vi "ST Step Joint.vi"(5 "error in (no error)":errorcluster, 6 "STEPS":string="1000", 7 "Combo Box":string(combo)="WAIST", 8 "VISA resource name":refnum<visa-resource-name>) -> (0 "error out":errorcluster, 1 "String Received":string, 2 "Ready and OK":bool, 3 "VISA resource name out":refnum<visa-resource-name>, 4 "Result Code":i32)   [LabVIEW 2009]
doc: "This VI will rotate a single joint, using joint mode. Select the joint to be rotated and the number of motor steps, - indicates reverse."
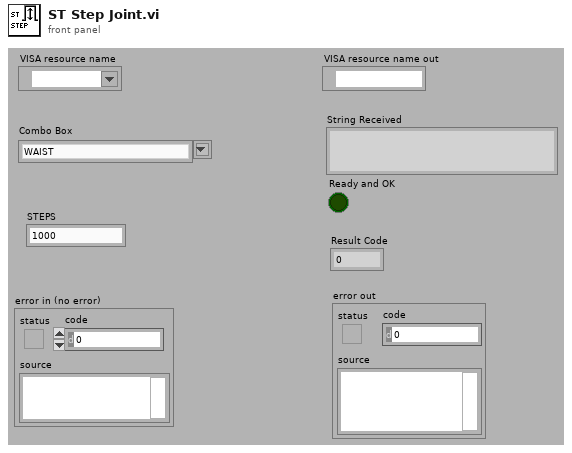
[diagram p1: front panel]
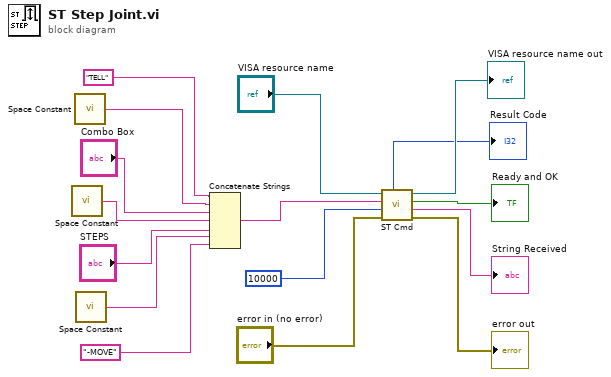
[diagram p0: block diagram]
diagram:
  n1 = call <vilib>:"Space Constant.vi"() -> ("String"=w4:string)
  n2 = call <vilib>:"Space Constant.vi"() -> ("String"=w6:string)
  n3 = call <vilib>:"Space Constant.vi"() -> ("String"=w1:string)
  n4 = Concatenate Strings("TELL", w6, "Combo Box", w4, "STEPS", w1, "-MOVE") -> (w7:string)
  n5 = call "ST Cmd.vi"("error in (no error)"="error in (no error)", "Time Out"=10000, "Command String"=w7, "VISA resource name"="VISA resource name") -> ("error out"=→"error out":errorcluster, "String Received"=→"String Received":string, "Ready and OK"=→"Ready and OK":bool, "VISA resource name out"=→"VISA resource name out":refnum<visa-resource-name>, "Result Code"=→"Result Code":i32)
